vi "snap test_continuous.vi"() -> ()   [LabVIEW 2013]
panel:
  out "ms between images":u32
  in  "stop":bool
  out "Image Out":T1(plugin-control)
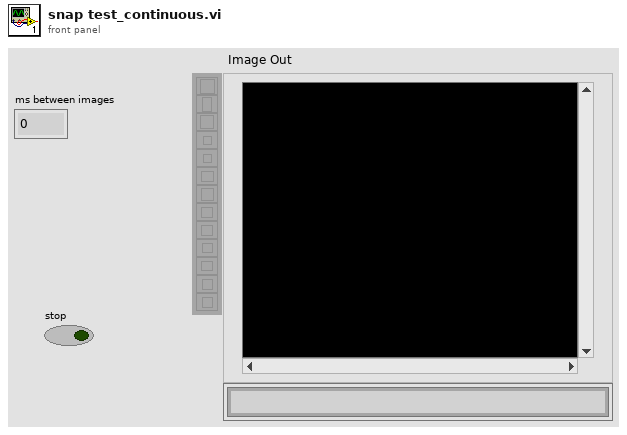
[diagram p1: front panel]
types:
  T1 = typedef "IMAQ Image.ctl" = refnum<image>
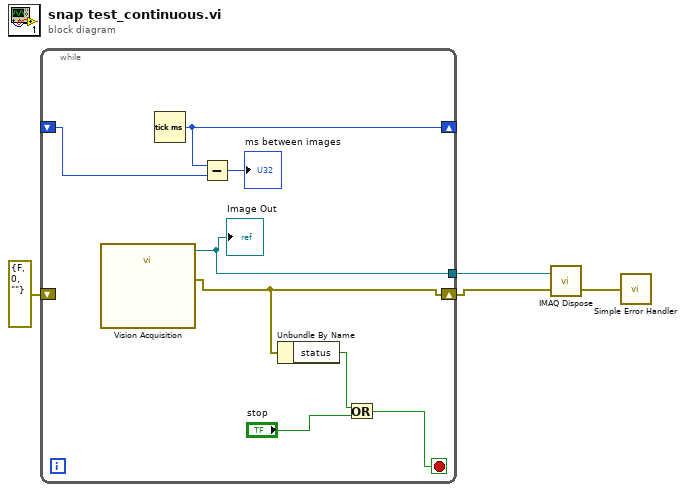
[diagram p0: block diagram]
diagram:
  n1 = while {
    tunnel: [w12] -> w4
    shift-right: [w8] -> w1
    shift-left: errorcluster {"status"=FALSE, "code"=0, "source"=""} ("error out") -> [_]
    shift-right: [w7] -> _
    shift-left: _ -> [w6]
    stop <- w9 stop-if-true
    n2 = call "Vision Acquisition"() -> ("Image Out"=w12:T1, "error out"=w8:errorcluster)  [unwired: 26 in]
    "Image Out" <- w12
    n3 = Tick Count (ms)() -> (millisecond timer value=w7:u32)
    n4 = Subtract(x=w7, y=w6) -> (x-y=→"ms between images":u32)
    n5 = Unbundle By Name(w8) -> ("status"=w11:bool)
    n6 = Or(x=w11, y="stop") -> (x .or. y?=w9:bool)
  }
  n7 = call "IMAQ Dispose"("Image"=w4, "error in (no error)"=w1) -> ("error out"=w3:errorcluster)  [unwired: 4 in]
  n8 = call <vilib>:"Simple Error Handler.vi"("error in (no error)"=w3) -> ()  [unwired: 4 in, 5 out]
